vi "Creat AO Chan.vi"(8 "error in (no error)":errorcluster caption="错误输入（无错误）", 11 "DAQ 输入":refnum<class "DAQ.lvclass">) -> (0 "error out":errorcluster caption="错误输出", 3 "DAQ 输出":refnum<class "DAQ.lvclass">)   [LabVIEW 2017, in "DAQ.lvlib" / "DAQ.lvclass"]
uses:
  DAQ.lvclass
  <vilib>/DAQmx/create/channels.llb/DAQmx Create Channel (AO-Voltage-Basic).vi
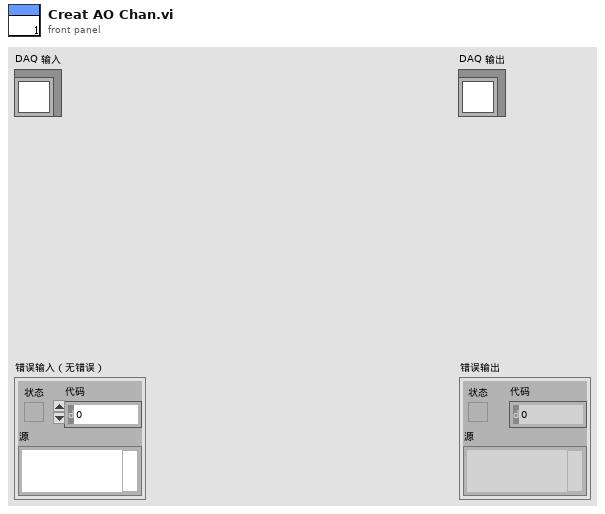
[diagram p1: front panel]
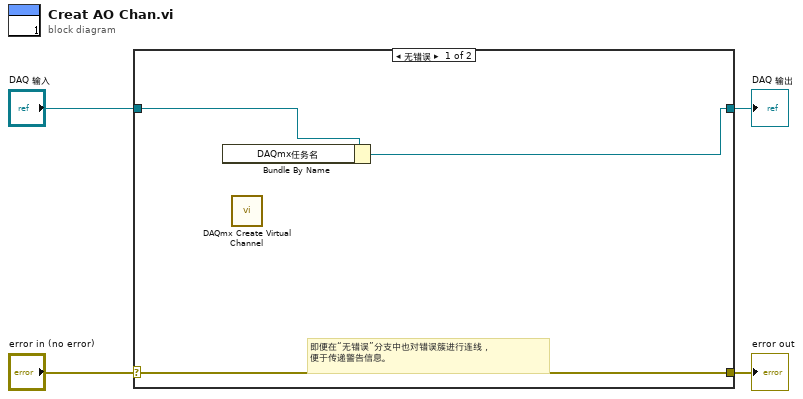
[diagram p0: block diagram]
diagram:
  n1 = case shown="无错误" "error in (no error)" {
    selector: "error in (no error)" -> [w7 w9]
    tunnel: [w7 w9] -> w3
    tunnel: [w5 w8] -> w1
    tunnel: "DAQ 输入" -> [w6 w8]
    frame No Error {
      # "即便在“无错误”分支中也对错误簇进行连线，\n便于传递警告信息。"
      n2 = Bundle By Name(cluster=w6) -> (w5:refnum<class "DAQ.lvclass">)  [unwired: 1 in]
      n3 = call-poly <vilib>:"DAQmx Create Virtual Channel.vi"() -> ()  [unwired: 14 in, 2 out]
    }
    frame Error {
    }
  }
  "error out" <- w3
  "DAQ 输出" <- w1
